vi "GananciasMotor.vi"() -> ()   [LabVIEW 2024]
uses:
  <vilib>/Instr/_visa.llb/VISA Configure Serial Port (Instr).vi
panel:
  in  "stop":bool
  out "read buffer":string
  in  "Dial":i32(knob) scale=0.0..360.0
  in  "baud rate (9600)":u32=9600
  in  "VISA resource name":refnum<visa-resource-name>
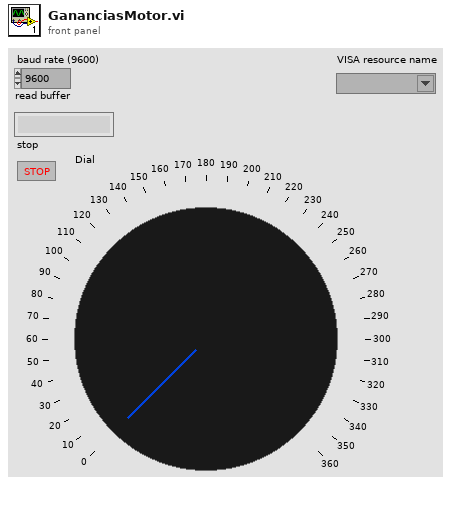
[diagram p1: front panel]
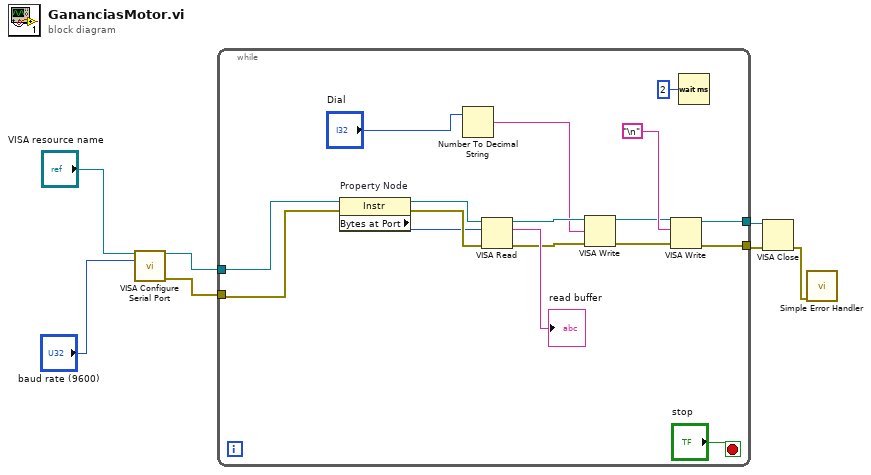
[diagram p0: block diagram]
diagram:
  n1 = call-poly "VISA Configure Serial Port"("VISA resource name"="VISA resource name", "baud rate (9600)"="baud rate (9600)") -> ("VISA resource name out"=w7:refnum<visa-resource-name>, "error out"=w6:errorcluster)  [unwired: 12 in]
  n2 = while {
    tunnel: w7 -> [w24]
    tunnel: w6 -> [w23]
    tunnel: [w13] -> w3
    tunnel: [w12] -> w2
    stop <- "stop" stop-if-true
    n3 = property on="Property Node" class="Instr"(reference=w24, error in=w23) -> (reference out=w10:refnum<visa-resource-name>, error out=w21:errorcluster, "Bytes at Port"=w8:u32)
    n4 = Number To Decimal String(number="Dial") -> (decimal integer string=w17:string)  [unwired: 1 in]
    n5 = VISA Read(VISA resource name=w10, byte count=w8, error in (no error)=w21) -> (VISA resource name out=w20:refnum<visa-resource-name>, read buffer=→"read buffer":string, error out=w19:errorcluster)  [unwired: 1 out]
    n6 = VISA Write(VISA resource name=w20, write buffer=w17, error in (no error)=w19) -> (VISA resource name out=w15:refnum<visa-resource-name>, error out=w14:errorcluster)  [unwired: 1 out]
    n7 = VISA Write(VISA resource name=w15, write buffer="\n", error in (no error)=w14) -> (VISA resource name out=w13:refnum<visa-resource-name>, error out=w12:errorcluster)  [unwired: 1 out]
    n8 = Wait (ms)(milliseconds to wait=u32 2) -> ()  [unwired: 1 out]
  }
  n9 = VISA Close(VISA resource name=w3, error in (no error)=w2) -> (error out=w1:errorcluster)
  n10 = call <vilib>:"Simple Error Handler.vi"("error in (no error)"=w1) -> ()  [unwired: 4 in, 5 out]
